vi "Close Report File.vi"(8 "error in (no error)":errorcluster, 11 "Mock Report In":refnum<class "Mock Report.lvclass">) -> (0 "error out":errorcluster)   [LabVIEW 2020, in "Mock Report.lvclass"]
uses:
  Mock Report.lvclass
  Mock Report.lvclass/Mock Report.ctl
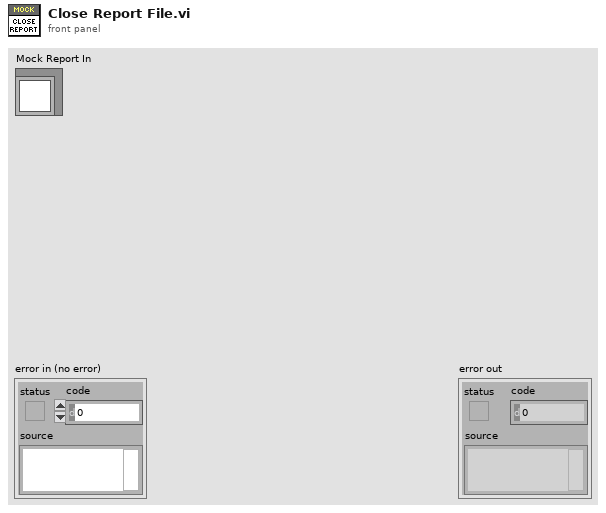
[diagram p1: front panel]
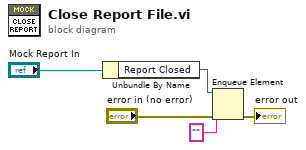
[diagram p0: block diagram]
diagram:
  n1 = Unbundle By Name("Mock Report In") -> ("Report Closed"=w2:refnum<queue>)
  n2 = Enqueue Element(queue=w2, element="", error in (no error)="error in (no error)") -> (error out=→"error out":errorcluster)  [unwired: 1 in, 2 out]
